vi "sub vi - temperature delay v4.vi"(8 "2-run":bool, 9 "1-run":bool, 10 "temp values IN":T1, 11 "temp signals":T2) -> (0 "T2-N":dbl, 1 "T2-L":dbl, 2 "T1-N":dbl, 3 "T1-L":dbl, 4 "temp values OUT":T1)   [LabVIEW 2017]
uses:
  Global 1.vi
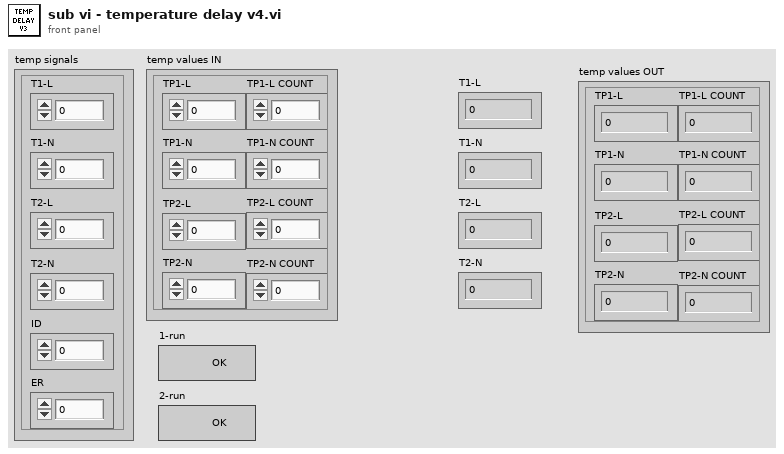
[diagram p1: front panel]
types:
  T1 = cluster{"TP1-L":dbl, "TP1-N":dbl, "TP2-L":dbl, "TP2-N":dbl, "TP1-L COUNT":dbl, "TP1-N COUNT":dbl, "TP2-L COUNT":dbl, "TP2-N COUNT":dbl}
  T2 = cluster{"T1-L":dbl, "T1-N":dbl, "T2-L":dbl, "T2-N":dbl, "ID":dbl, "ER":dbl}
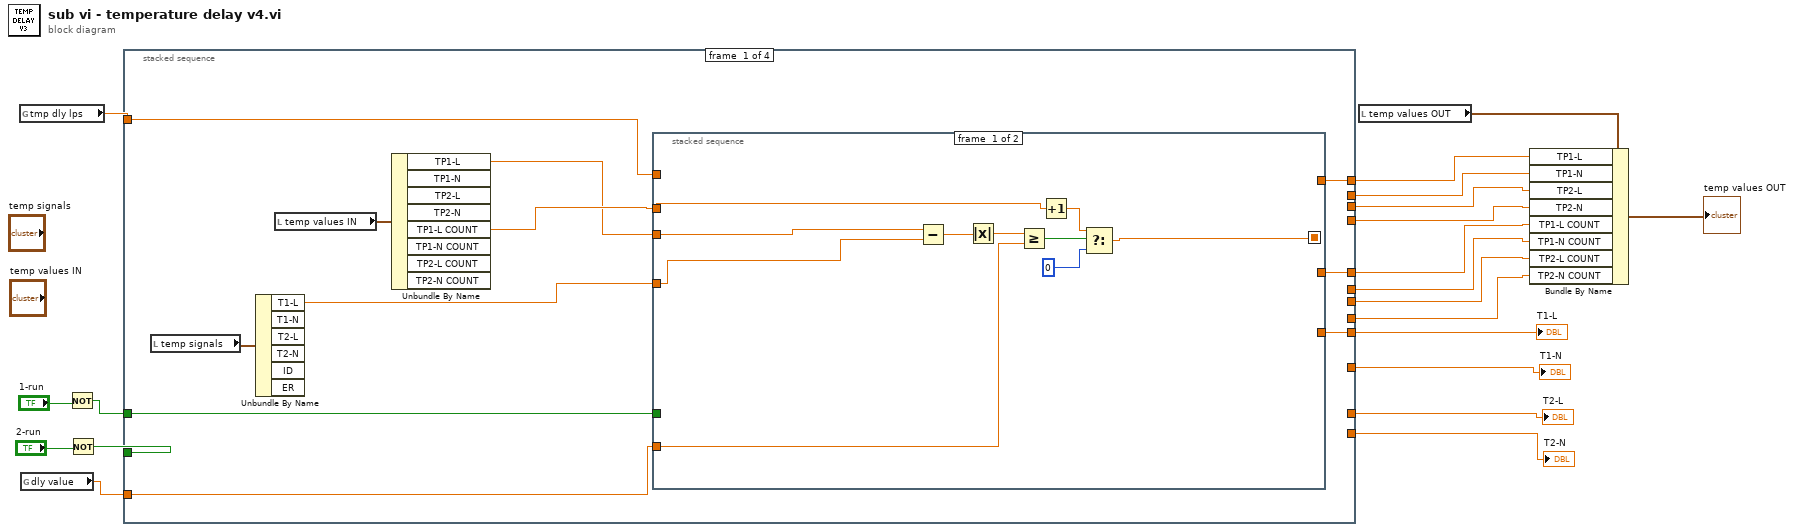
[diagram p0: block diagram]
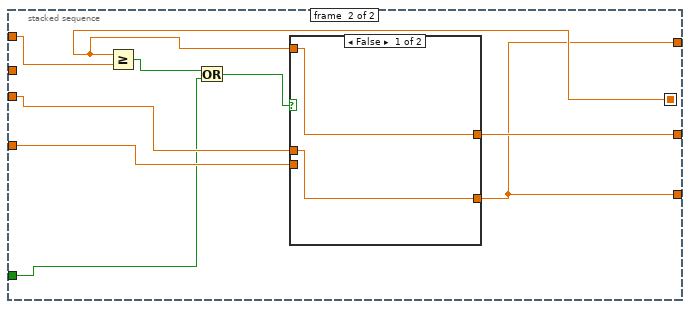
[diagram p2: hidden frame]
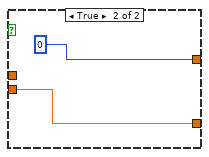
[diagram p3: hidden frame]
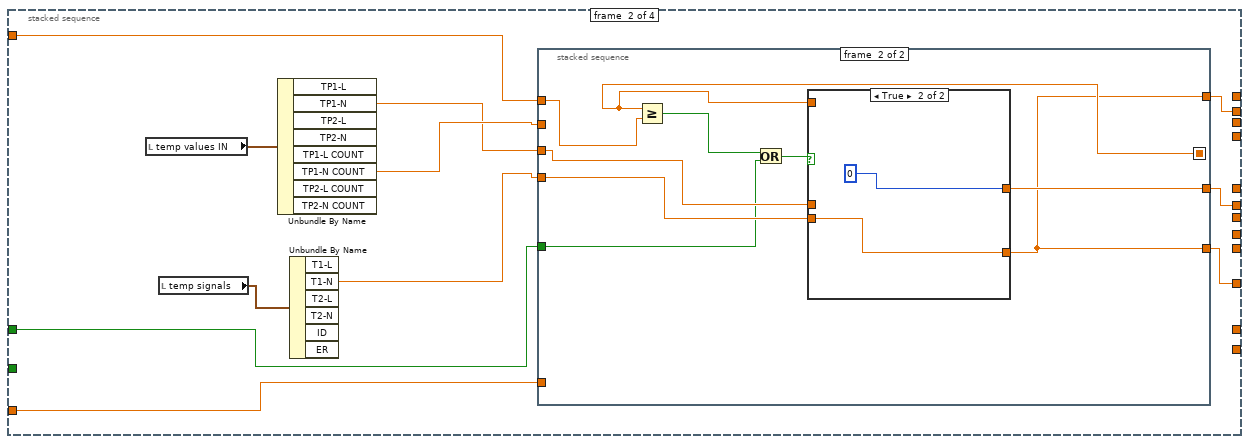
[diagram p4: hidden frame]
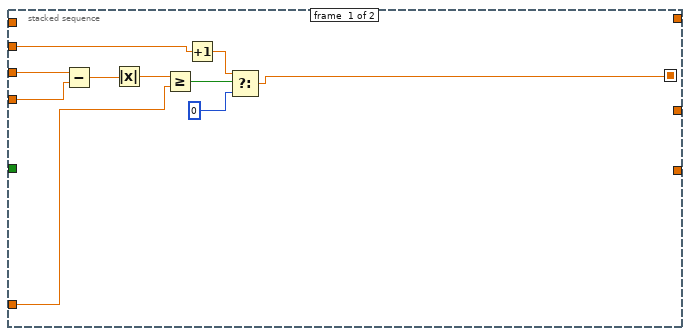
[diagram p5: hidden frame]
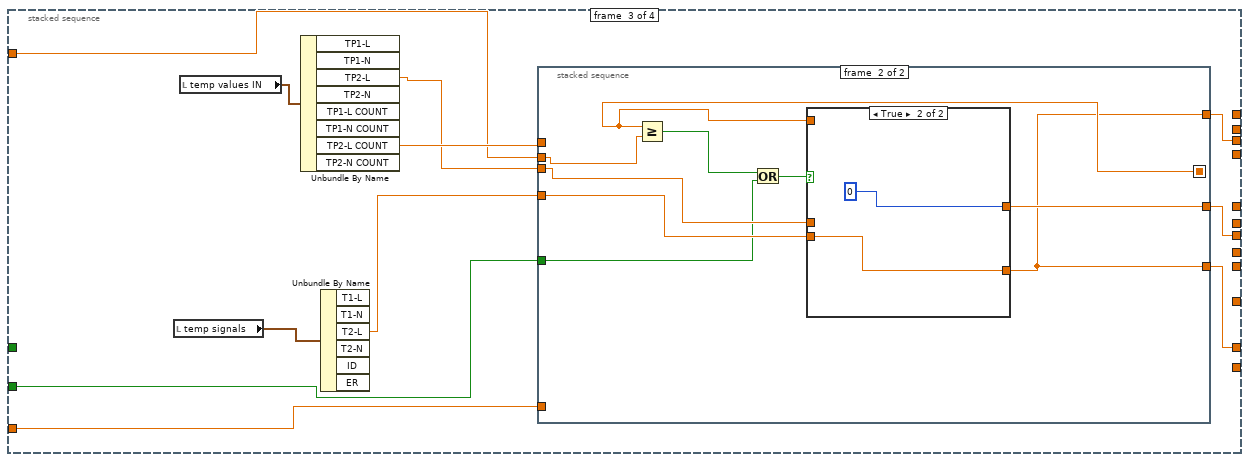
[diagram p7: hidden frame]
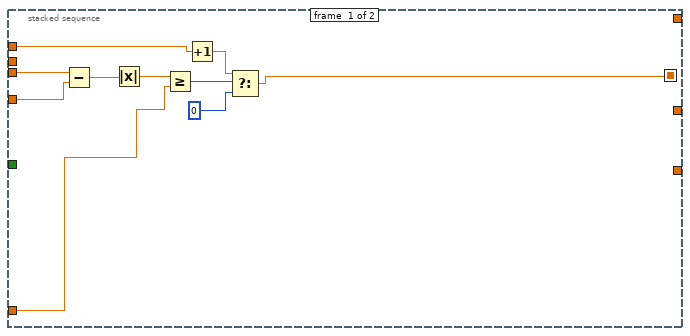
[diagram p8: hidden frame]
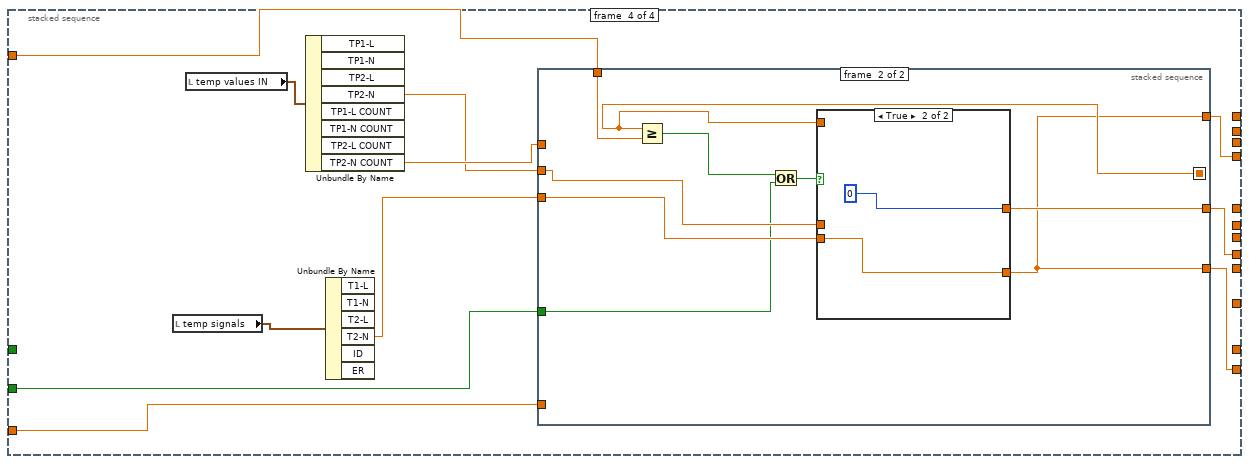
[diagram p10: hidden frame]
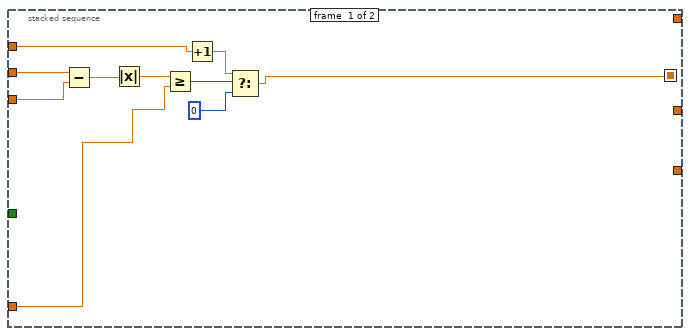
[diagram p11: hidden frame]
diagram:
  n1 = global read "Global 1.vi" "tmp dly lps"() -> (w6:dbl)
  n2 = global read "Global 1.vi" "dly value"() -> (w5:dbl)
  n3 = Not(x="1-run") -> (.not. x?=w2:bool)
  n4 = Not(x="2-run") -> (.not. x?=w1:bool)
  n5 = stacked-sequence {
    tunnel: [w31 _ _ _] -> w18
    tunnel: [w30 _ _ _] -> w17
    tunnel: [w29 _ _ _] -> w16
    tunnel: [_ w65 _ _] -> w15
    tunnel: [_ w64 _ _] -> w14
    tunnel: [_ w63 _ _] -> w13
    tunnel: [_ _ w99 _] -> w12
    tunnel: [_ _ w98 _] -> w11
    tunnel: [_ _ w97 _] -> w10
    tunnel: [_ _ _ w133] -> w9
    tunnel: [_ _ _ w132] -> w8
    tunnel: [_ _ _ w131] -> w7
    tunnel: w6 -> [w24 w56 w90 w124]
    tunnel: w5 -> [w23 w57 w91 w125]
    tunnel: w2 -> [w22 w55 _ _]
    tunnel: w1 -> [_ _ w89 w123]
    frame #0 {
      n6 = local read "temp signals"() -> (w28:T2)
      n7 = Unbundle By Name(w28) -> ("T1-L"=w21:dbl)  [unwired: 5 out]
      n8 = local read "temp values IN"() -> (w27:T1)
      n9 = Unbundle By Name(w27) -> ("TP1-L"=w25:dbl, "TP1-L COUNT"=w26:dbl)  [unwired: 6 out]
      n10 = stacked-sequence {
        seq-local: [w35 _] -> [_ w47]
        tunnel: w25 -> [w33 w49]
        tunnel: w21 -> [w32 w50]
        tunnel: w26 -> [w36 _]
        tunnel: [_ w48] -> w31
        tunnel: [_ w46] -> w30
        tunnel: [_ w46] -> w29
        tunnel: w23 -> [w34 _]
        tunnel: w24 -> [_ w45]
        tunnel: w22 -> [_ w43]
        frame #0 {
          n11 = Subtract(x=w33, y=w32) -> (x-y=w41:dbl)
          n12 = Absolute Value(x=w41) -> (abs(x)=w40:dbl)
          n13 = Greater Or Equal?(x=w40, y=w34) -> (x >= y?=w39:bool)
          n14 = Increment(x=w36) -> (x+1=w38:dbl)
          n15 = Select(t=w38, s=w39, f=0) -> (s? t:f=w35:dbl)
        }
        frame #1 {
          n16 = Greater Or Equal?(x=w47, y=w45) -> (x >= y?=w44:bool)
          n17 = Or(x=w44, y=w43) -> (x .or. y?=w42:bool)
          n18 = case shown="False" w42 {
            tunnel: [w52 w54] -> w46
            tunnel: w50 -> [_ w54]
            tunnel: w49 -> [w52 _]
            tunnel: [w51 0] -> w48
            tunnel: w47 -> [w51 _]
            frame False {
            }
            frame True {
            }
          }
        }
      }
    }
    frame #1 {
      n19 = local read "temp values IN"() -> (w62:T1)
      n20 = local read "temp signals"() -> (w59:T2)
      n21 = Unbundle By Name(w62) -> ("TP1-N"=w60:dbl, "TP1-N COUNT"=w61:dbl)  [unwired: 6 out]
      n22 = Unbundle By Name(w59) -> ("T1-N"=w58:dbl)  [unwired: 5 out]
      n23 = stacked-sequence {
        seq-local: [w67 _] -> [_ w81]
        tunnel: w60 -> [w70 w83]
        tunnel: w58 -> [w69 w84]
        tunnel: w61 -> [w68 _]
        tunnel: [_ w82] -> w64
        tunnel: [_ w80] -> w65
        tunnel: [_ w80] -> w63
        tunnel: w57 -> [w66 _]
        tunnel: w56 -> [_ w79]
        tunnel: w55 -> [_ w76]
        frame #0 {
          n24 = Subtract(x=w70, y=w69) -> (x-y=w75:dbl)
          n25 = Absolute Value(x=w75) -> (abs(x)=w74:dbl)
          n26 = Greater Or Equal?(x=w74, y=w66) -> (x >= y?=w73:bool)
          n27 = Increment(x=w68) -> (x+1=w72:dbl)
          n28 = Select(t=w72, s=w73, f=0) -> (s? t:f=w67:dbl)
        }
        frame #1 {
          n29 = Greater Or Equal?(x=w81, y=w79) -> (x >= y?=w77:bool)
          n30 = Or(x=w77, y=w76) -> (x .or. y?=w78:bool)
          n31 = case shown="True" w78 {
            tunnel: [w86 w88] -> w80
            tunnel: w84 -> [_ w88]
            tunnel: w83 -> [w86 _]
            tunnel: [w85 0] -> w82
            tunnel: w81 -> [w85 _]
            frame False {
            }
            frame True {
            }
          }
        }
      }
    }
    frame #2 {
      n32 = local read "temp signals"() -> (w95:T2)
      n33 = local read "temp values IN"() -> (w96:T1)
      n34 = Unbundle By Name(w96) -> ("TP2-L"=w93:dbl, "TP2-L COUNT"=w94:dbl)  [unwired: 6 out]
      n35 = Unbundle By Name(w95) -> ("T2-L"=w92:dbl)  [unwired: 5 out]
      n36 = stacked-sequence {
        seq-local: [w101 _] -> [_ w115]
        tunnel: w93 -> [w104 w117]
        tunnel: w92 -> [w103 w118]
        tunnel: w94 -> [w102 _]
        tunnel: [_ w116] -> w98
        tunnel: [_ w114] -> w99
        tunnel: [_ w114] -> w97
        tunnel: w91 -> [w100 _]
        tunnel: w90 -> [_ w113]
        tunnel: w89 -> [_ w110]
        frame #0 {
          n37 = Subtract(x=w104, y=w103) -> (x-y=w109:dbl)
          n38 = Absolute Value(x=w109) -> (abs(x)=w108:dbl)
          n39 = Greater Or Equal?(x=w108, y=w100) -> (x >= y?=w107:bool)
          n40 = Increment(x=w102) -> (x+1=w106:dbl)
          n41 = Select(t=w106, s=w107, f=0) -> (s? t:f=w101:dbl)
        }
        frame #1 {
          n42 = Greater Or Equal?(x=w115, y=w113) -> (x >= y?=w111:bool)
          n43 = Or(x=w111, y=w110) -> (x .or. y?=w112:bool)
          n44 = case shown="True" w112 {
            tunnel: [w120 w122] -> w114
            tunnel: w118 -> [_ w122]
            tunnel: w117 -> [w120 _]
            tunnel: [w119 0] -> w116
            tunnel: w115 -> [w119 _]
            frame False {
            }
            frame True {
            }
          }
        }
      }
    }
    frame #3 {
      n45 = local read "temp signals"() -> (w130:T2)
      n46 = local read "temp values IN"() -> (w129:T1)
      n47 = Unbundle By Name(w129) -> ("TP2-N"=w127:dbl, "TP2-N COUNT"=w128:dbl)  [unwired: 6 out]
      n48 = Unbundle By Name(w130) -> ("T2-N"=w126:dbl)  [unwired: 5 out]
      n49 = stacked-sequence {
        seq-local: [w135 _] -> [_ w149]
        tunnel: w127 -> [w138 w151]
        tunnel: w126 -> [w137 w152]
        tunnel: w128 -> [w136 _]
        tunnel: [_ w150] -> w132
        tunnel: [_ w148] -> w133
        tunnel: [_ w148] -> w131
        tunnel: w125 -> [w134 _]
        tunnel: w124 -> [_ w147]
        tunnel: w123 -> [_ w144]
        frame #0 {
          n50 = Subtract(x=w138, y=w137) -> (x-y=w143:dbl)
          n51 = Absolute Value(x=w143) -> (abs(x)=w142:dbl)
          n52 = Greater Or Equal?(x=w142, y=w134) -> (x >= y?=w141:bool)
          n53 = Increment(x=w136) -> (x+1=w140:dbl)
          n54 = Select(t=w140, s=w141, f=0) -> (s? t:f=w135:dbl)
        }
        frame #1 {
          n55 = Greater Or Equal?(x=w149, y=w147) -> (x >= y?=w145:bool)
          n56 = Or(x=w145, y=w144) -> (x .or. y?=w146:bool)
          n57 = case shown="True" w146 {
            tunnel: [w154 w156] -> w148
            tunnel: w152 -> [_ w156]
            tunnel: w151 -> [w154 _]
            tunnel: [w153 0] -> w150
            tunnel: w149 -> [w153 _]
            frame False {
            }
            frame True {
            }
          }
        }
      }
    }
  }
  "T1-N" <- w13
  "T2-L" <- w10
  "T2-N" <- w7
  "T1-L" <- w16
  n58 = local read "temp values OUT"() -> (w20:T1)
  n59 = Bundle By Name(cluster=w20, "TP1-L"=w17, "TP1-N"=w15, "TP2-L"=w12, "TP2-N"=w9, "TP1-L COUNT"=w18, "TP1-N COUNT"=w14, "TP2-L COUNT"=w11, "TP2-N COUNT"=w8) -> (→"temp values OUT":T1)
